vi "Save_meas_data_MOA.vi"(0 "Path":path, 5 "Meas. Param. Data Cluster":T2, 7 "Data":T1, 11 "error in":errorcluster) -> (15 "error out":errorcluster)   [LabVIEW 2018]
uses:
  Data_MOA.ctl
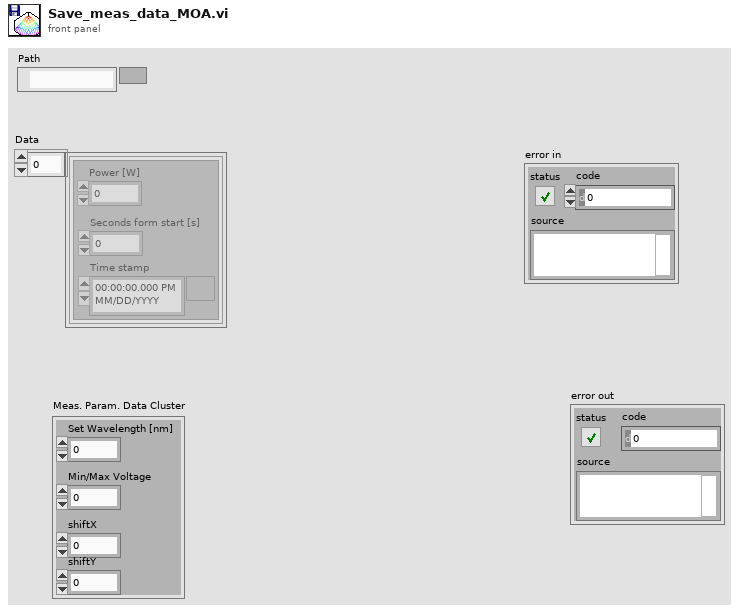
[diagram p1: front panel]
types:
  T1 = typedef "Data_MOA.ctl" = cluster{cluster{"Power [W]":dbl, "Seconds form start [s]":dbl, "Time stamp":timestamp}}[]
  T2 = cluster{"Set Wavelength [nm]":dbl, "Min/Max Voltage":dbl, "shiftX":dbl, "shiftY":dbl}
  T3 = enum16{"open", "replace", "create", "open or create", "replace or create", "replace or create with confirmation"}
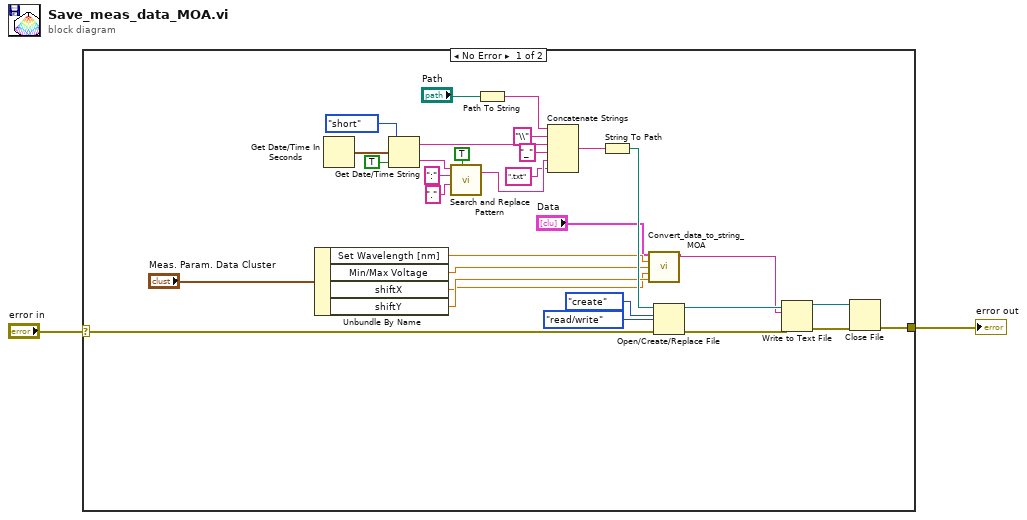
[diagram p0: block diagram]
diagram:
  n1 = case shown="No Error" "error in" {
    selector: "error in" -> [w10 w34]
    tunnel: [w33 w34] -> w2
    frame No Error {
      n2 = Unbundle By Name("Meas. Param. Data Cluster") -> ("Set Wavelength [nm]"=w4:dbl, "Min/Max Voltage"=w5:dbl, "shiftX"=w6:dbl, "shiftY"=w7:dbl)
      n3 = Get Date/Time In Seconds() -> (seconds since 1Jan1904=w12:timestamp)
      n4 = Get Date/Time String(date format (0)=enum16{"short", "long", "abbreviated"}."short", seconds (now)=w12, want seconds? (F)=TRUE) -> (date string=w15:string, time string=w31:string)
      n5 = call <vilib>:"Search and Replace Pattern.vi"("string"=w31, "regular expression (\"\")"=":" ("regular expression (\"\")"), "replace string (\"\")"="." ("replace string (\"\")"), "replace all? (F)"=TRUE) -> ("result string"=w30:string)  [unwired: 1 in, 1 out]
      n6 = Path To String(path="Path") -> (string=w23:string)
      n7 = Concatenate Strings(w23, "\\" ("string"), w15, "_", w30, ".txt" ("string")) -> (w21:string)
      n8 = String To Path(string=w21) -> (path=w25:path)
      n9 = call "Convert_data_to_string_MOA.vi"("Data"="Data", "Wavelenght [nm]"=w4, "Min/Max Voltage [V]"=w5, "X Shift [V]"=w6, "Y Shift [V]"=w7) -> ("spreadsheet string"=w8:string)  [unwired: 10 in]
      n10 = Open/Create/Replace File(file path (use dialog)=w25, error in=w10, operation (0:open)=T3."create", access (0:read/write)=enum16{"read/write", "read-only", "write-only"}."read/write") -> (refnum out=w17:refnum<file>, error out=w26:errorcluster)  [unwired: 2 in, 1 out]
      n11 = Write to Text File(file (use dialog)=w17, text=w8, error in=w26) -> (refnum out=w11:refnum<file>, error out=w27:errorcluster)  [unwired: 1 in, 1 out]
      n12 = Close File(refnum=w11, error in=w27) -> (error out=w33:errorcluster)  [unwired: 1 out]
    }
    frame Error {
    }
  }
  "error out" <- w2
